vi "Cluster.vi"() -> ()   [LabVIEW 2015]
panel:
  out "Cluster":T1
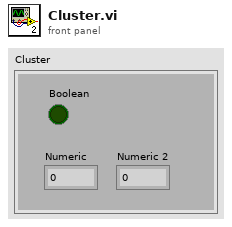
[diagram p1: front panel]
types:
  T1 = cluster{"Boolean":bool, "Numeric":dbl, "Numeric 2":dbl}
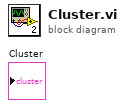
[diagram p0: block diagram]
diagram:
